vi "CfgManager.Text.INI (Array) Test Launcher.vi"() -> ()   [LabVIEW 2013]
uses:
  source/Manager.Text.INI/ConfigManager.Text.INI.lvclass
  source/Manager/Decompose KVPs.vi
  source/Manager/Write.vi
  source/Manager/ConfigManager.lvclass
panel:
  out "_dyndependencies":T1(array[cluster])
  out "Keys":string[](array[string])
  out "error out":errorcluster
  out "filepath":path
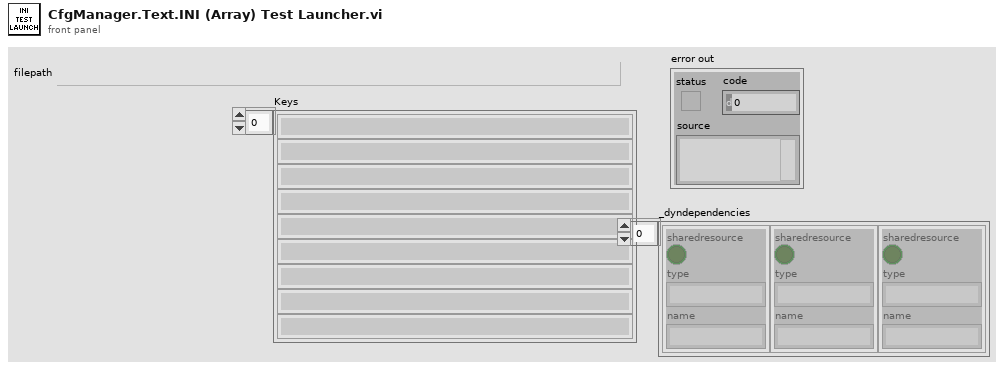
[diagram p1: front panel]
types:
  T1 = cluster{"sharedresource":bool, "type":string, "name":string}[]
  T2 = cluster{"sharedresource":bool, "type":string, "name":string}
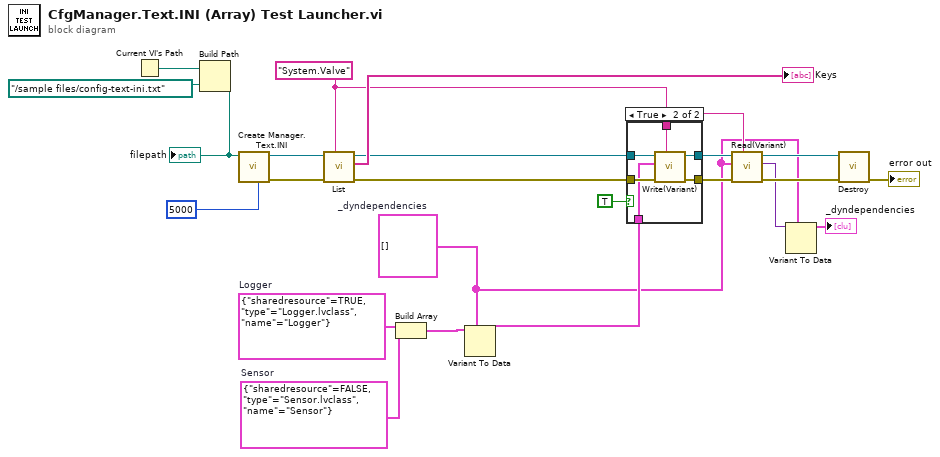
[diagram p0: block diagram]
diagram:
  w2 = T1 []  # _dyndependencies
  w14 = T2 {"sharedresource"=FALSE, "type"="Sensor.lvclass", "name"="Sensor"}  # Sensor
  w15 = T2 {"sharedresource"=TRUE, "type"="Logger.lvclass", "name"="Logger"}  # Logger
  w4 = "System.Valve" ("Qualified Name")
  n1 = Current VI's Path() -> (path=w21:path)
  n2 = Build Path(base path=w21, name or relative path=path "../sample files/config-text-ini.txt" ("filepath 2")) -> (appended path=w19:path)
  "filepath" <- w19
  n3 = call "Create Manager.Text.INI.vi"("write delay (ms)"=5000, "filepath"=w19) -> ("error out"=w17:errorcluster, "ConfigManager.Text.INI out"=w18:refnum<class "ConfigManager.Text.INI.lvclass">)  [unwired: 7 in, 1 out]
  n4 = call "List.vi"("Qualified Name"=w4, "error in (no error)"=w17, "ConfigManager in"=w18) -> ("error out"=w5:errorcluster, "Keys"=→"Keys":string[], "ConfigManager out"=w6:refnum<class "ConfigManager.Text.INI.lvclass">)  [unwired: 6 in]
  n5 = Build Array(w15, w14) -> (w1:T1)
  n6 = Variant To Data(type=w2, Variant=w1) -> (data=w13:T1)  [unwired: 1 in, 1 out]
  n7 = case shown="True" TRUE {
    tunnel: w6 -> [w25 w31]
    tunnel: w5 -> [w24 w30]
    tunnel: w13 -> [_ w29]
    tunnel: [w25 w28] -> w12
    tunnel: [w24 w27] -> w10
    tunnel: w4 -> [_ w26]
    frame False {
    }
    frame True {
      n8 = call "Write(Variant).vi"("Qualified Name"=w26, "error in (no error)"=w30, "value"=w29, "ConfigManager in"=w31) -> ("error out"=w27:errorcluster, "ConfigManager out"=w28:refnum<class "ConfigManager.Text.INI.lvclass">)  [unwired: 5 in, 1 out]
    }
  }
  n9 = call "Read(Variant).vi"("Qualified Name"=w4, "error in (no error)"=w10, "Type"=w2, "ConfigManager in"=w12) -> ("error out"=w9:errorcluster, "value"=w8:variant, "ConfigManager out"=w11:refnum<class "ConfigManager.Text.INI.lvclass">)  [unwired: 3 in, 2 out]
  n10 = Variant To Data(type=w2, Variant=w8) -> (data=→"_dyndependencies":T1)  [unwired: 1 in, 1 out]
  n11 = call-dynamic "Destroy.vi"("error in (no error)"=w9, "ConfigManager.Text in"=w11) -> ("error out"=→"error out":errorcluster)  [unwired: 8 in, 1 out]
